vi "Update Column Headers.vi"(8 "error in (no error)":errorcluster, 11 "List Box View Model in":refnum<class "Process Tree View Model.lvclass">) -> (0 "error out":errorcluster, 3 "List Box View Model out":refnum<class "Process Tree View Model.lvclass">)   [LabVIEW 2020, in "Process Tree View Model.lvclass"]
uses:
  Process Tree View Model.lvclass
  Process Tree View Model.lvclass/Process Tree View Model.ctl
  Tree Helpers/Tag Tree/Tag Tree.lvclass
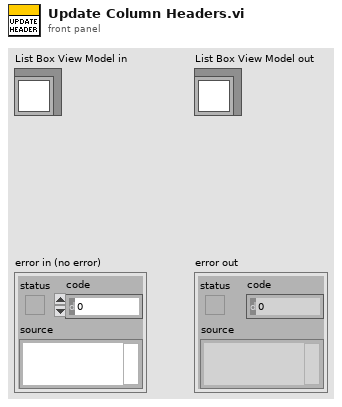
[diagram p1: front panel]
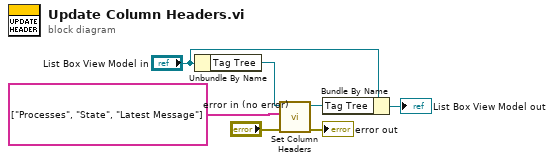
[diagram p0: block diagram]
diagram:
  n1 = Unbundle By Name("List Box View Model in") -> ("Tag Tree"=w6:refnum<class "Tag Tree.lvclass">)
  n2 = call "Set Column Headers.vi"("error in (no error)"="error in (no error)", "Column Header Strings[]"=string[] ["Processes", "State", "Latest Message"], "Tag Tree in"=w6) -> ("error out"=→"error out":errorcluster, "Tag Tree out"=w3:refnum<class "Tag Tree.lvclass">)  [unwired: 7 in]
  n3 = Bundle By Name(cluster="List Box View Model in", "Tag Tree"=w3) -> (→"List Box View Model out":refnum<class "Process Tree View Model.lvclass">)
